vi "WriteTDMS.vi"(0 "object in":refnum<class "Experiment.lvclass">, 1 "Pump Array":T2(array[cluster]), 2 "FileNames":string[](array[string]), 3 "Array of timestamps":dbl[](array[numeric]), 5 "error in (no error)":errorcluster, 9 "Coriolis Data":T1) -> (14 "object out":refnum<class "Experiment.lvclass">, 19 "error out":errorcluster)   [LabVIEW 2021, in "Experiment.lvclass"]
uses:
  Experiment.lvclass
  Experiment.lvclass/Experiment.ctl
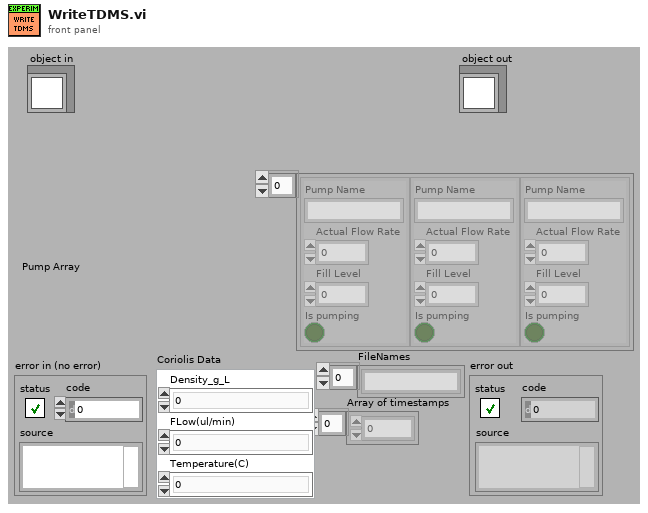
[diagram p1: front panel]
types:
  T1 = cluster{"Density_g_L":sgl, "FLow(ul/min)":sgl, "Temperature(C)":sgl}
  T2 = cluster{"Pump Name":string, "Actual Flow Rate":dbl, "Fill Level":dbl, "Is pumping":bool}[]
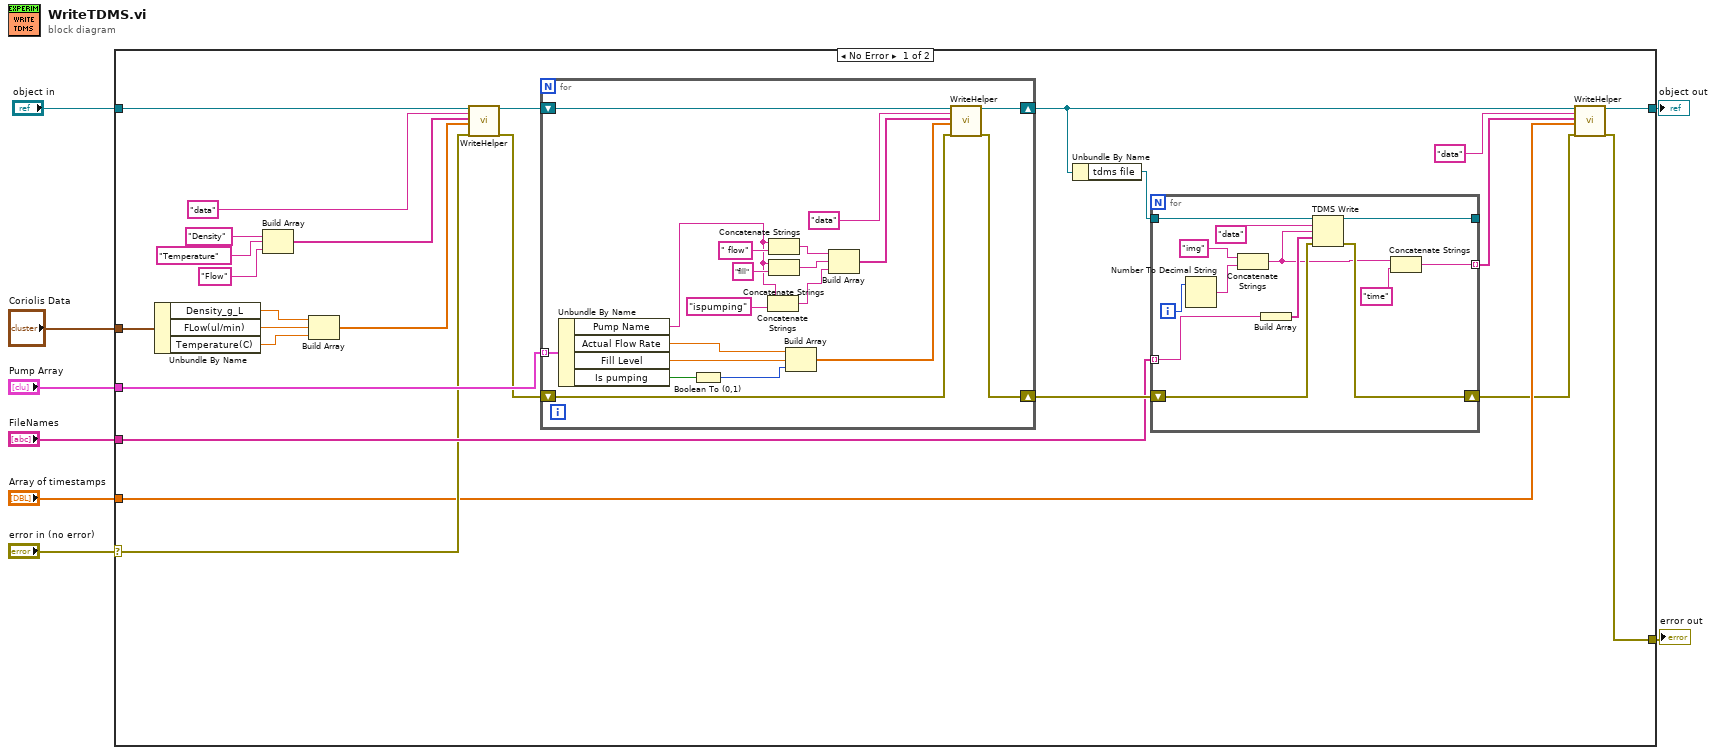
[diagram p0: block diagram]
diagram:
  n1 = case shown="No Error" "error in (no error)" {
    selector: "error in (no error)" -> [w20 w67]
    tunnel: [w14 w67] -> w7
    tunnel: [w12 w66] -> w5
    tunnel: "object in" -> [w9 w66]
    tunnel: "Coriolis Data" -> [w28 _]
    tunnel: "Pump Array" -> [w27 _]
    tunnel: "Array of timestamps" -> [w16 _]
    tunnel: "FileNames" -> [w26 _]
    frame No Error {
      n2 = Unbundle By Name(w28) -> ("Density_g_L"=w24:sgl, "FLow(ul/min)"=w30:sgl, "Temperature(C)"=w29:sgl)
      n3 = Build Array("Density" ("group name in (Untitled)"), "Temperature" ("group name in (Untitled)"), "Flow" ("group name in (Untitled)")) -> (w22:string[])
      n4 = Build Array(w24, w30, w29) -> (w21:sgl[])
      n5 = call-dynamic "WriteHelper.vi"("object in"=w9, "Group name"="data" ("group name in (Untitled)"), "Channel Names"=w22, "Data array"=w21, "error in (no error)"=w20) -> ("object out"=w10:refnum<class "Experiment.lvclass">, "error out"=w19:errorcluster)  [unwired: 13 in]
      n6 = for {
        tunnel: w27 -> [w65] mode=indexing
        shift-right: [w49] -> w31
        shift-left: w19 -> [w50]
        shift-right: [w47] -> w11
        shift-left: w10 -> [w48]
        n7 = Unbundle By Name(w65) -> ("Pump Name"=w59:string, "Actual Flow Rate"=w63:dbl, "Fill Level"=w64:dbl, "Is pumping"=w58:bool)
        n8 = Boolean To (0,1)(Boolean=w58) -> (0, 1=w57:i16)
        n9 = Concatenate Strings(w59, "ispumping" ("string")) -> (w54:string)
        n10 = Concatenate Strings(w59, " flow" ("string")) -> (w56:string)
        n11 = Concatenate Strings(w59, "fill" ("string")) -> (w55:string)
        n12 = Build Array(w63, w64, w57) -> (w51:dbl[])
        n13 = Build Array(w56, w55, w54) -> (w52:string[])
        n14 = call-dynamic "WriteHelper.vi"("object in"=w48, "Group name"="data" ("group name in (Untitled)"), "Channel Names"=w52, "Data array"=w51, "error in (no error)"=w50) -> ("object out"=w47:refnum<class "Experiment.lvclass">, "error out"=w49:errorcluster)  [unwired: 13 in]
      }
      n15 = Unbundle By Name(w11) -> ("tdms file"=w13:refnum<k34>)
      n16 = for {
        tunnel: w26 -> [w42] mode=indexing
        tunnel: w13 -> [w43]
        shift-right: [w36] -> w15
        shift-left: w31 -> [w40]
        tunnel: [w38] -> w17 mode=indexing
        tunnel: [w37] -> _
        i -> [w46]
        n17 = Number To Decimal String(number=w46) -> (decimal integer string=w45:string)  [unwired: 1 in]
        n18 = Concatenate Strings("img" ("string"), w45) -> (w34:string)
        n19 = Build Array(w42) -> (w41:string[])
        n20 = TDMS Write(0:w43, 5:"data" ("group name in (Untitled)"), 7:w34, 9:w41, 11:w40) -> (4:w37:refnum<k34>, 15:w36:errorcluster)  [unwired: 1 in, 2 out]
        n21 = Concatenate Strings(w34, "time" ("string")) -> (w38:string)
      }
      n22 = call-dynamic "WriteHelper.vi"("object in"=w11, "Group name"="data" ("group name in (Untitled)"), "Channel Names"=w17, "Data array"=w16, "error in (no error)"=w15) -> ("object out"=w12:refnum<class "Experiment.lvclass">, "error out"=w14:errorcluster)  [unwired: 13 in]
    }
    frame Error {
    }
  }
  "error out" <- w7
  "object out" <- w5
